vi "VI Tree.vi"   [LabVIEW 2012, in "Phidget Common.lvlib"]
doc: "This is the instrument driver for the Phidget Common library. The VI Tree displays all the user-callable VIs of the instrument driver in an organized table."
uses:
  <instrlib>/Phidgets/Phidget Common/Phidget Common.lvlib
  <instrlib>/Phidgets/Phidget RC Servo/Phidget RC Servo.lvlib
  <instrlib>/Phidgets/Phidget Temperature Sensor/Phidget Temperature Sensor.lvlib
panel:
  # "(c) 2015 Phidgets Inc..  ALL RIGHTS RESERVED."
  # "SEE DIAGRAM\nFOR VI TREE."
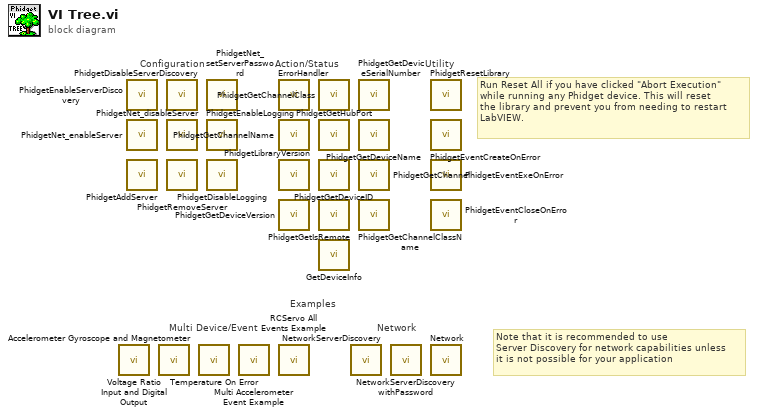
[diagram p0: block diagram]
diagram:
  # "Note that it is recommended to use\nServer Discovery for network capabilities unless\nit is not possible for your application"
  # "Network"
  # "Multi Device/Event"
  # "Examples"
  # "Run Reset All if you have clicked \"Abort Execution\"\nwhile running any Phidget device. This will reset\nthe library and prevent you from needing to restart\nLabVIEW."
  # "Configuration"
  # "Utility"
  # "Action/Status"
  n1 = call <instrlib>:"Voltage Ratio Input and Digital Output.vi"() -> ()  [unwired: 12 in]
  n2 = call <instrlib>:"PhidgetEnableServerDiscovery.vi"() -> ()  [unwired: 11 in, 1 out]
  n3 = call <instrlib>:"PhidgetNet_enableServer.vi"() -> ()  [unwired: 11 in, 1 out]
  n4 = call <instrlib>:"PhidgetAddServer.vi"() -> ()  [unwired: 11 in, 1 out]
  n5 = call <instrlib>:"Accelerometer Gyroscope and Magnetometer.vi"() -> ()  [unwired: 12 in]
  n6 = call <instrlib>:"PhidgetDisableServerDiscovery.vi"() -> ()  [unwired: 11 in, 1 out]
  n7 = call <instrlib>:"PhidgetNet_disableServer.vi"() -> ()  [unwired: 11 in, 1 out]
  n8 = call <instrlib>:"PhidgetRemoveServer.vi"() -> ()  [unwired: 11 in, 1 out]
  n9 = call <instrlib>:"Temperature On Error.vi"() -> ()  [unwired: 12 in]
  n10 = call <instrlib>:"PhidgetNet_setServerPassword.vi"() -> ()  [unwired: 11 in, 1 out]
  n11 = call <instrlib>:"PhidgetEnableLogging.vi"() -> ()  [unwired: 11 in, 1 out]
  n12 = call <instrlib>:"PhidgetDisableLogging.vi"() -> ()  [unwired: 11 in, 1 out]
  n13 = call <instrlib>:"Multi Accelerometer Event Example.vi"() -> ()  [unwired: 12 in]
  n14 = call <instrlib>:"ErrorHandler.vi"() -> ()  [unwired: 10 in, 2 out]
  n15 = call <instrlib>:"PhidgetGetChannelName.vi"() -> ()  [unwired: 9 in, 3 out]
  n16 = call <instrlib>:"PhidgetLibraryVersion.vi"() -> ()  [unwired: 10 in, 2 out]
  n17 = call <instrlib>:"PhidgetGetDeviceVersion.vi"() -> ()  [unwired: 9 in, 3 out]
  n18 = call <instrlib>:"RCServo All Events Example.vi"() -> ()  [unwired: 12 in]
  n19 = call <instrlib>:"PhidgetGetChannelClass.vi"() -> ()  [unwired: 8 in, 3 out]
  n20 = call <instrlib>:"PhidgetGetHubPort.vi"() -> ()  [unwired: 9 in, 3 out]
  n21 = call <instrlib>:"PhidgetGetDeviceID.vi"() -> ()  [unwired: 8 in, 3 out]
  n22 = call <instrlib>:"PhidgetGetIsRemote.vi"() -> ()  [unwired: 8 in, 3 out]
  n23 = call <instrlib>:"GetDeviceInfo.vi"() -> ()  [unwired: 6 in, 6 out]
  n24 = call <instrlib>:"NetworkServerDiscovery.vi"() -> ()  [unwired: 12 in]
  n25 = call <instrlib>:"PhidgetGetDeviceSerialNumber.vi"() -> ()  [unwired: 9 in, 3 out]
  n26 = call <instrlib>:"PhidgetGetDeviceName.vi"() -> ()  [unwired: 9 in, 3 out]
  n27 = call <instrlib>:"PhidgetGetChannel.vi"() -> ()  [unwired: 8 in, 3 out]
  n28 = call <instrlib>:"PhidgetGetChannelClassName.vi"() -> ()  [unwired: 9 in, 3 out]
  n29 = call <instrlib>:"NetworkServerDiscoverywithPassword.vi"() -> ()  [unwired: 12 in]
  n30 = call <instrlib>:"PhidgetResetLibrary.vi"() -> ()  [unwired: 11 in, 1 out]
  n31 = call <instrlib>:"PhidgetEventCreateOnError.vi"() -> ()  [unwired: 9 in, 3 out]
  n32 = call <instrlib>:"PhidgetEventExeOnError.vi"() -> ()  [unwired: 8 in, 8 out]
  n33 = call <instrlib>:"PhidgetEventCloseOnError.vi"() -> ()  [unwired: 10 in, 2 out]
  n34 = call <instrlib>:"Network.vi"() -> ()  [unwired: 12 in]
